vi "DependencyFilter.vi"(9 "FilterOptions":T1, 11 "LibraryDependency In":map{path, T2}(c390)) -> (3 "Filtered LibraryDependency Out":map{path, T2}(c390))   [LabVIEW 2020, in "DependencyViewer.lvlib"]
uses:
  DependencyViewer/DependencyViewer.lvlib
  LibraryDependentInfo.vi
  <vilib>/Utility/lvfile.llb/FT_FileTypes.ctl
  FilterOptions.ctl
  <vilib>/Utility/lvfile.llb/NI_FileType.lvlib
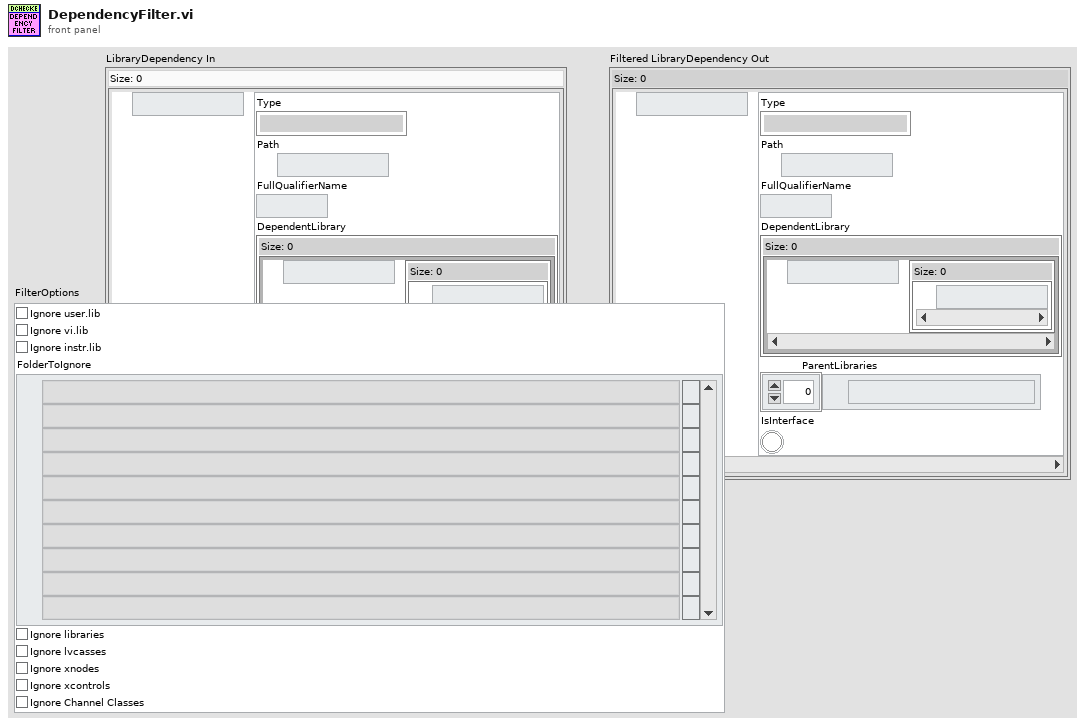
[diagram p1: front panel]
types:
  T1 = typedef "DependencyViewer.lvlib/FilterOptions.ctl" = cluster{"Ignore user.lib":bool, "Ignore vi.lib":bool, "Ignore instr.lib":bool, "FolderToIgnore":path[], "Ignore libraries":bool, "Ignore lvcasses":bool, "Ignore xnodes":bool, "Ignore xcontrols":bool, "Ignore Channel Classes":bool}
  T2 = typedef "DependencyViewer.lvlib/LibraryDependentInfo.vi" = cluster{"Type":T3, "Path":path, "FullQualifierName":string, "DependentLibrary":map{path, set{path}}, "ParentLibraries":path[], "IsInterface":bool}
  T3 = typedef "NI_FileType.lvlib/FT_FileTypes.ctl" = enum32{"Invalid file/path", "Unknown type", "Instrument", "Control", "Polymorphic VI", "Project", "Library", "LVClass", "XControl", "XNode", "CIN", "Run-time menu", "Palette menu", "LLB", "Shortcut", "Directory", "Class Private Data Control", "Statechart", "MathScript .m file", "Ladder Diagram", "LVLibp"}
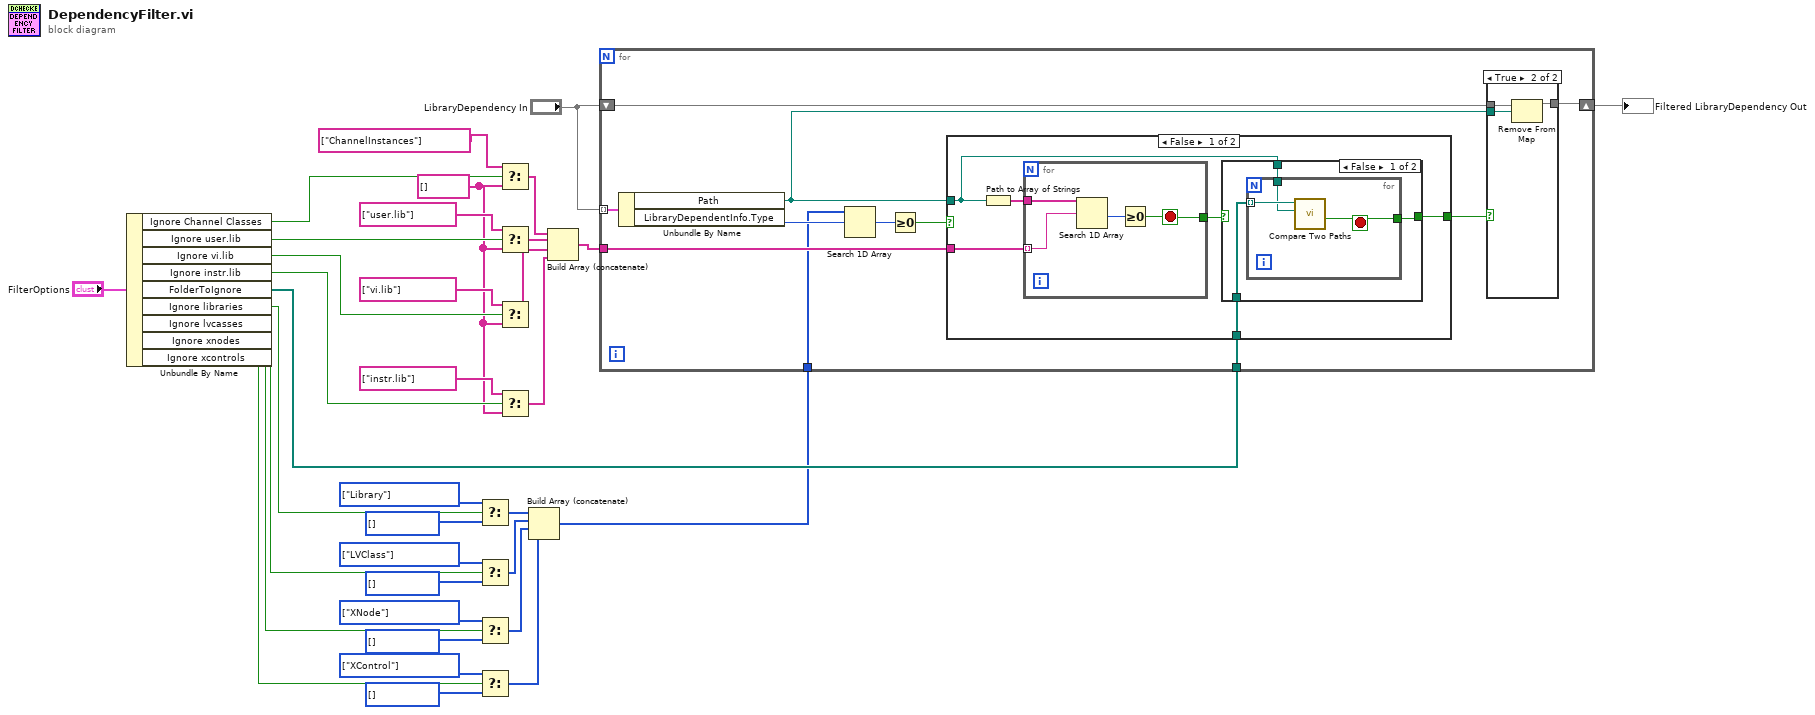
[diagram p0: block diagram]
diagram:
  w14 = T3[] [] items=["Invalid file/path", "Unknown type", "Instrument", "Control", "Polymorphic VI", "Project", "Library", "LVClass", "XControl", "XNode", "CIN", "Run-time menu", "Palette menu", "LLB", "Shortcut", "Directory", "Class Private Data Control", "Statechart", "MathScript .m file", "Ladder Diagram", "LVLibp"] ("f")
  w13 = T3[] [enum."XControl"] items=["Invalid file/path", "Unknown type", "Instrument", "Control", "Polymorphic VI", "Project", "Library", "LVClass", "XControl", "XNode", "CIN", "Run-time menu", "Palette menu", "LLB", "Shortcut", "Directory", "Class Private Data Control", "Statechart", "MathScript .m file", "Ladder Diagram", "LVLibp"] ("1D array")
  w15 = T3[] [] items=["Invalid file/path", "Unknown type", "Instrument", "Control", "Polymorphic VI", "Project", "Library", "LVClass", "XControl", "XNode", "CIN", "Run-time menu", "Palette menu", "LLB", "Shortcut", "Directory", "Class Private Data Control", "Statechart", "MathScript .m file", "Ladder Diagram", "LVLibp"] ("f")
  w16 = T3[] [enum."XNode"] items=["Invalid file/path", "Unknown type", "Instrument", "Control", "Polymorphic VI", "Project", "Library", "LVClass", "XControl", "XNode", "CIN", "Run-time menu", "Palette menu", "LLB", "Shortcut", "Directory", "Class Private Data Control", "Statechart", "MathScript .m file", "Ladder Diagram", "LVLibp"] ("1D array")
  w18 = T3[] [] items=["Invalid file/path", "Unknown type", "Instrument", "Control", "Polymorphic VI", "Project", "Library", "LVClass", "XControl", "XNode", "CIN", "Run-time menu", "Palette menu", "LLB", "Shortcut", "Directory", "Class Private Data Control", "Statechart", "MathScript .m file", "Ladder Diagram", "LVLibp"] ("f")
  w17 = T3[] [enum."LVClass"] items=["Invalid file/path", "Unknown type", "Instrument", "Control", "Polymorphic VI", "Project", "Library", "LVClass", "XControl", "XNode", "CIN", "Run-time menu", "Palette menu", "LLB", "Shortcut", "Directory", "Class Private Data Control", "Statechart", "MathScript .m file", "Ladder Diagram", "LVLibp"] ("1D array")
  w20 = T3[] [] items=["Invalid file/path", "Unknown type", "Instrument", "Control", "Polymorphic VI", "Project", "Library", "LVClass", "XControl", "XNode", "CIN", "Run-time menu", "Palette menu", "LLB", "Shortcut", "Directory", "Class Private Data Control", "Statechart", "MathScript .m file", "Ladder Diagram", "LVLibp"] ("f")
  w21 = T3[] [enum."Library"] items=["Invalid file/path", "Unknown type", "Instrument", "Control", "Polymorphic VI", "Project", "Library", "LVClass", "XControl", "XNode", "CIN", "Run-time menu", "Palette menu", "LLB", "Shortcut", "Directory", "Class Private Data Control", "Statechart", "MathScript .m file", "Ladder Diagram", "LVLibp"] ("1D array")
  w3 = string[] [] ("f")
  n1 = Unbundle By Name("FilterOptions") -> ("Ignore Channel Classes"=w4:bool, "Ignore user.lib"=w34:bool, "Ignore vi.lib"=w30:bool, "Ignore instr.lib"=w29:bool, "FolderToIgnore"=w24:path[], "Ignore libraries"=w22:bool, "Ignore lvcasses"=w12:bool, "Ignore xnodes"=w11:bool, "Ignore xcontrols"=w10:bool)
  n2 = Select(t=w21, s=w22, f=w20) -> (s? t:f=w19:T3[])
  n3 = Select(t=w17, s=w12, f=w18) -> (s? t:f=w9:T3[])
  n4 = Select(t=w16, s=w11, f=w15) -> (s? t:f=w8:T3[])
  n5 = Select(t=w13, s=w10, f=w14) -> (s? t:f=w7:T3[])
  n6 = Select(t=string[] ["ChannelInstances"], s=w4, f=w3) -> (s? t:f=w1:string[])
  n7 = Select(t=string[] ["user.lib"], s=w34, f=w3) -> (s? t:f=w28:string[])
  n8 = Select(t=string[] ["vi.lib"], s=w30, f=w3) -> (s? t:f=w27:string[])
  n9 = Select(t=string[] ["instr.lib"], s=w29, f=w3) -> (s? t:f=w26:string[])
  n10 = Build Array (concatenate)(w19, w9, w8, w7) -> (w6:T3[])
  n11 = Build Array (concatenate)(w1, w28, w27, w26) -> (w25:string[])
  n12 = for {
    tunnel: "LibraryDependency In" -> [w46] mode=indexing
    shift-right: [w43] -> w23
    shift-left: "LibraryDependency In" -> [w44]
    tunnel: w25 -> [w45]
    tunnel: w24 -> [w42]
    tunnel: w6 -> [w39]
    n13 = Unbundle By Name(w46) -> ("Path"=w41:path, "LibraryDependentInfo.Type"=w40:T3)
    n14 = Search 1D Array(1D array=w39, element=w40) -> (index of element=w38:i32)  [unwired: 1 in]
    n15 = Greater Or Equal To 0?(x=w38) -> (x >= 0?=w36:bool)
    n16 = case shown="False" w36 {
      selector: w36 -> [_ w64]
      tunnel: w45 -> [w52 _]
      tunnel: w42 -> [w51 _]
      tunnel: w41 -> [w50 _]
      tunnel: [w47 w64] -> w37
      frame False {
        n17 = Path to Array of Strings(0:w50) -> (2:w49:string[])  [unwired: 1 out]
        n18 = for {
          tunnel: w49 -> [w63]
          tunnel: w52 -> [w62] mode=indexing
          tunnel: [w60] -> w48
          stop <- w60 stop-if-true
          n19 = Search 1D Array(1D array=w63, element=w62) -> (index of element=w61:i32)  [unwired: 1 in]
          n20 = Greater Or Equal To 0?(x=w61) -> (x >= 0?=w60:bool)
        }
        n21 = case shown="False" w48 {
          selector: w48 -> [_ w59]
          tunnel: [w53 w59] -> w47
          tunnel: w51 -> [w55 _]
          tunnel: w50 -> [w54 _]
          frame False {
            n22 = for {
              tunnel: w55 -> [w58] mode=indexing
              tunnel: w54 -> [w57]
              tunnel: [w56] -> w53
              stop <- w56 stop-if-true
              n23 = call <vilib>:"Compare Two Paths.vi"("Path 2"=w57, "Path 1"=w58) -> ("Path 2 Relative to Path 1?"=w56:bool)  [unwired: 6 in, 3 out]
            }
          }
          frame True {
          }
        }
      }
      frame True {
      }
    }
    n24 = case shown="True" w37 {
      tunnel: w44 -> [w65 w68]
      tunnel: w41 -> [_ w67]
      tunnel: [w65 w66] -> w43
      frame False {
      }
      frame True {
        n25 = Remove From Map(10:w67, 11:w68) -> (3:w66:map{path, T2})  [unwired: 2 out]
      }
    }
  }
  "Filtered LibraryDependency Out" <- w23
